vi "Find_Nearest_Dot_in_Next_Frm_less_dRmin.vi"(0 "X":dbl, 1 "Y":dbl, 2 "dR min":dbl, 3 "n+1 frame\ncolumn (X,Y)":dbl[](array[numeric]), 4 "Max number\nof dots in \ncolumn (X,Y)":i32) -> (5 "Any dots found?":bool, 6 "index of the dot \nwith minimal displ":i32)   [LabVIEW 2013]
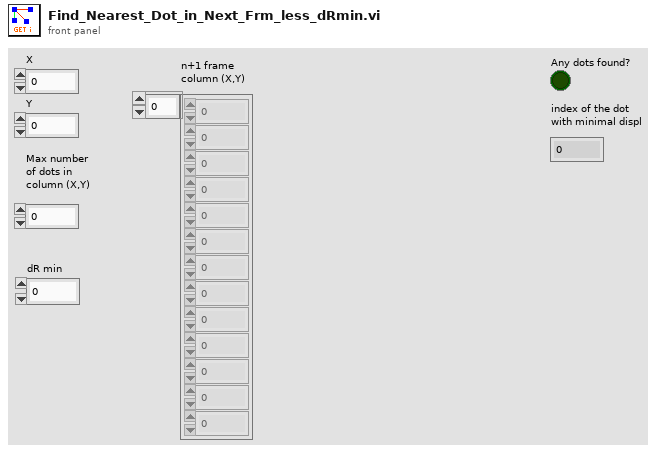
[diagram p1: front panel]
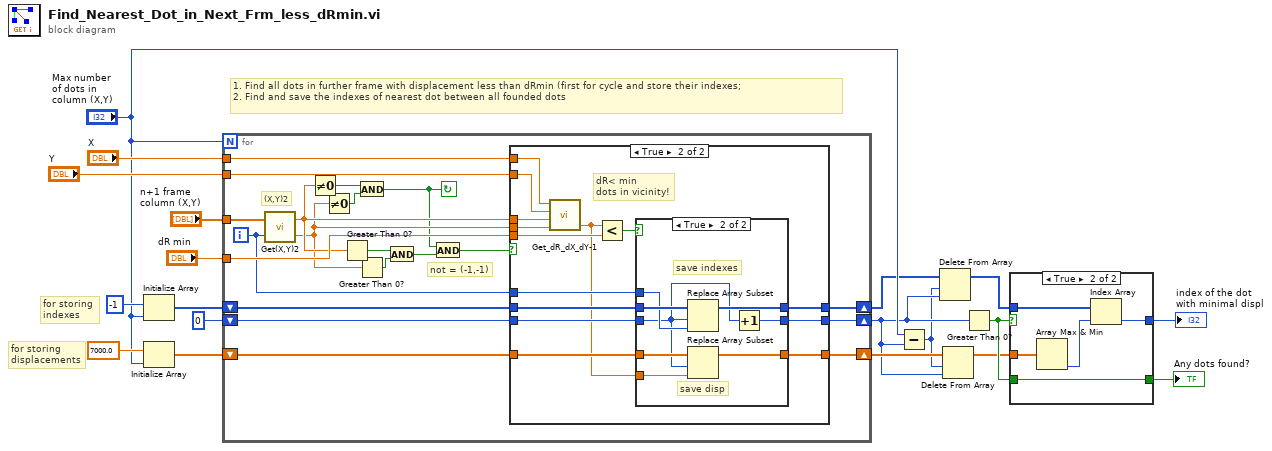
[diagram p0: block diagram]
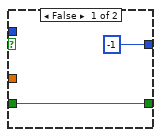
[diagram p2: hidden frame]
diagram:
  # "for storing\ndisplacements"
  # "for storing\nindexes"
  # "1. Find all dots in further frame with displacement less than dRmin (first for cycle and store their indexes;\n2. Find and save the indexes of nearest dot between all founded dots"
  n1 = Initialize Array(-1, "Max number\nof dots in \ncolumn (X,Y)") -> (w14:i32[])
  n2 = Initialize Array(7000.0 ("element"), "Max number\nof dots in \ncolumn (X,Y)") -> (w12:dbl[])
  n3 = for {
    N: "Max number\nof dots in \ncolumn (X,Y)" -> [_]
    tunnel: "X" -> [w36]
    tunnel: "Y" -> [w35]
    tunnel: "n+1 frame\ncolumn (X,Y)" -> [w39]
    tunnel: "dR min" -> [w34]
    shift-right: [w23] -> w4
    shift-left: w14 -> [w26]
    shift-right: [w22] -> w3
    shift-left: 0 -> [w25]
    shift-right: [w20] -> w7
    shift-left: w12 -> [w21]
    i -> [w24]
    stop <- w27 continue-if-true
    # "not = (-1,-1)"
    # "(X,Y)2"
    n4 = call "Get(X,Y)2.vi"("[IN] index of (X,Y)"=w24, "[IN] Array coordi\nnates (X,Y) in Frame"=w39) -> ("[OUT] Y"=w28:dbl, "[OUT] X"=w29:dbl)
    n5 = Not Equal To 0?(x=w29) -> (x != 0?=w37:bool)
    n6 = Not Equal To 0?(x=w28) -> (x != 0?=w38:bool)
    n7 = Greater Than 0?(x=w29) -> (x > 0?=w32:bool)
    n8 = And(x=w37, y=w38) -> (x .and. y?=w27:bool)
    n9 = Greater Than 0?(x=w28) -> (x > 0?=w33:bool)
    n10 = And(x=w32, y=w33) -> (x .and. y?=w30:bool)
    n11 = And(x=w27, y=w30) -> (x .and. y?=w31:bool)
    n12 = case shown="True" w31 {
      tunnel: w36 -> [_ w56]
      tunnel: w35 -> [_ w55]
      tunnel: w29 -> [_ w52]
      tunnel: w28 -> [_ w51]
      tunnel: w34 -> [_ w54]
      tunnel: w26 -> [w42 w50]
      tunnel: w25 -> [w41 w49]
      tunnel: w24 -> [_ w48]
      tunnel: [w42 w47] -> w23
      tunnel: [w41 w46] -> w22
      tunnel: w21 -> [w40 w45]
      tunnel: [w40 w43] -> w20
      frame False {
      }
      frame True {
        # "dR< min\ndots in vicinity!"
        n13 = call "Get_dR_dX_dY-1.vi"("Y2"=w51, "X2"=w52, "Y1"=w55, "X1"=w56) -> ("dR"=w44:dbl)  [unwired: 2 out]
        n14 = Less?(x=w44, y=w54) -> (x < y?=w53:bool)
        n15 = case shown="True" w53 {
          tunnel: w50 -> [w59 w67]
          tunnel: w49 -> [w57 w60]
          tunnel: w48 -> [_ w61]
          tunnel: [w59 w66] -> w47
          tunnel: [w57 w65] -> w46
          tunnel: w45 -> [w58 w63]
          tunnel: w44 -> [_ w64]
          tunnel: [w58 w62] -> w43
          frame False {
          }
          frame True {
            # "save indexes"
            # "save disp"
            n16 = Replace Array Subset(array=w67, new element=w61, index=w60) -> (w66:i32[])
            n17 = Replace Array Subset(array=w63, new element=w64, index=w60) -> (w62:dbl[])
            n18 = Increment(x=w60) -> (x+1=w65:i32)
          }
        }
      }
    }
  }
  n19 = Subtract(x="Max number\nof dots in \ncolumn (X,Y)", y=w3) -> (x-y=w2:i32)
  n20 = Delete From Array(array=w4, length=w2, index=w3) -> (array with subset deleted=w1:i32[])  [unwired: 1 out]
  n21 = Delete From Array(array=w7, length=w2, index=w3) -> (array with subset deleted=w6:dbl[])  [unwired: 1 out]
  n22 = Greater Than 0?(x=w3) -> (x > 0?=w11:bool)
  n23 = case shown="True" w11 {
    tunnel: w6 -> [_ w74]
    tunnel: w1 -> [_ w73]
    tunnel: w11 -> [w69 w70]
    tunnel: [w69 w70] -> w10
    tunnel: [-1 w71] -> w9
    frame False {
    }
    frame True {
      n24 = Array Max & Min(array=w74) -> (min index (indices)=w72:i32)  [unwired: 3 out]
      n25 = Index Array(array=w73, index=w72) -> (element=w71:i32)
    }
  }
  "Any dots found?" <- w10
  "index of the dot \nwith minimal displ" <- w9
